vi "使用例子.vi"() -> ()   [LabVIEW 2015, in "PLC.lvlib"]
uses:
  PLC.lvlib
panel:
  in  "端口选择":refnum<visa-resource-name>="COM3"
  in  "波特率":u32(ring)=9600 items=["9600"=9600, "19200"=19200, "115200"=115200]
  in  "校检":u32(ring)=2 items=["无", "偶", "奇"]
  in  "数据位":u32(ring)=7 items=["7"=7, "8"=8]
  in  "16位/32位":u32(ring) items=["16bit", "32bit"]
  in  "写入":bool
  in  "写入数据":string
  in  "PLC地址":string="0"
  in  "变量类型":u32(ring)=2 items=["X", "Y", "M", "D"]
  out "读取数据输出":u32
  in  "读出":bool
  in  "M7":bool
  in  "M6":bool
  in  "M5":bool
  in  "M4":bool
  in  "M3":bool
  in  "M2":bool
  in  "M1":bool
  in  "M0":bool
  # "数据取值范围"
  # "寻址范围"
  # "X0-X577"
  # "0或1"
  # "Y0-Y577"
  # "0或1"
  # "M0-M7999"
  # "0或1"
  # "D0-D7999"
  # "16bit或32bit"
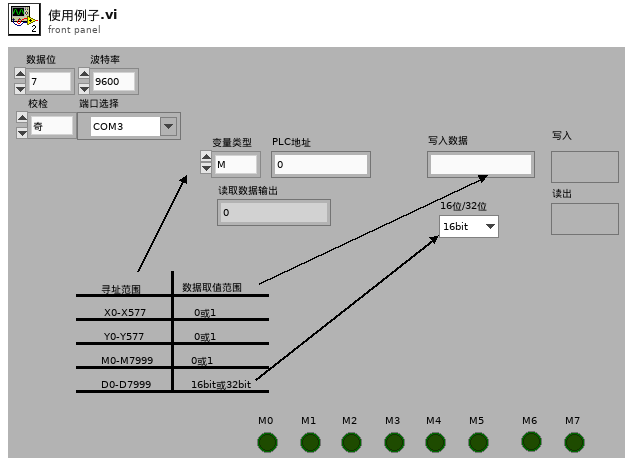
[diagram p1: front panel]
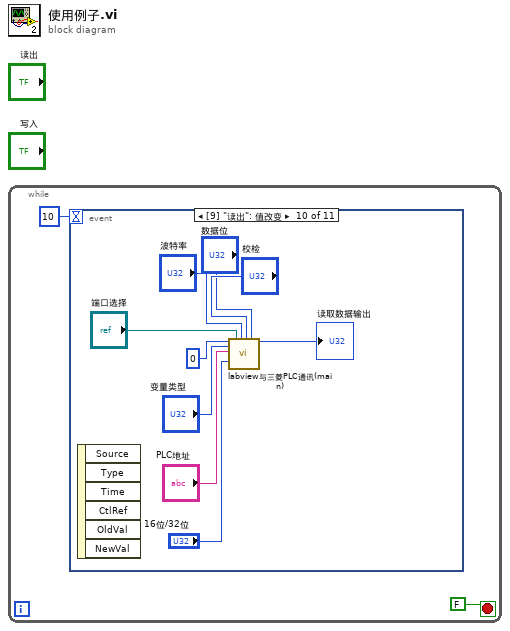
[diagram p0: block diagram]
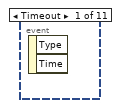
[diagram p2: hidden frame]
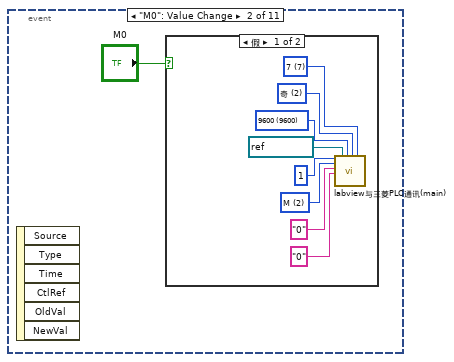
[diagram p3: hidden frame]
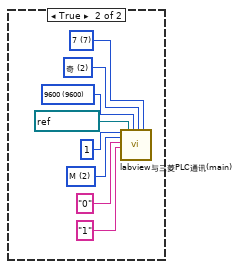
[diagram p4: hidden frame]
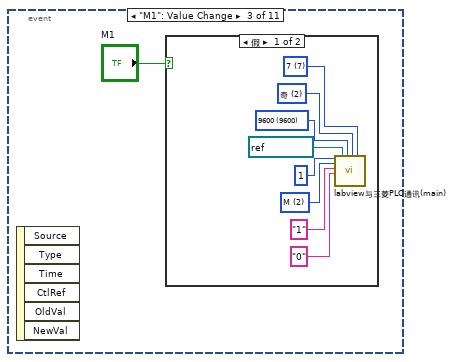
[diagram p5: hidden frame]
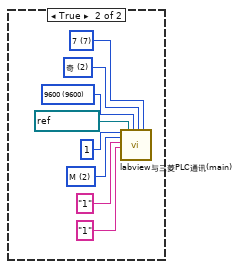
[diagram p6: hidden frame]
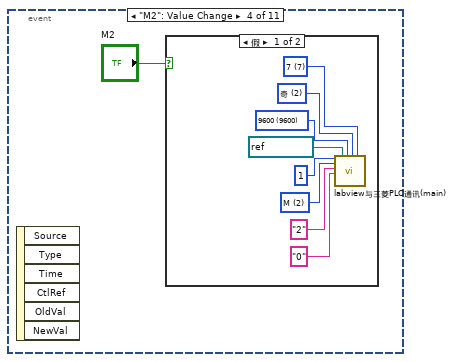
[diagram p7: hidden frame]
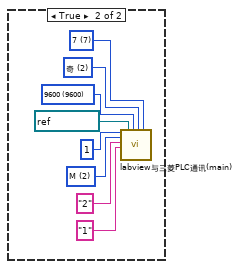
[diagram p8: hidden frame]
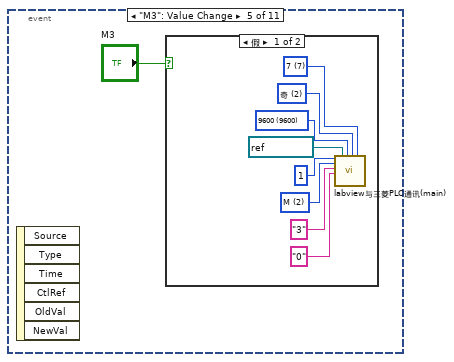
[diagram p9: hidden frame]
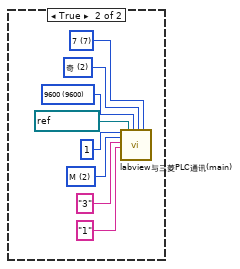
[diagram p10: hidden frame]
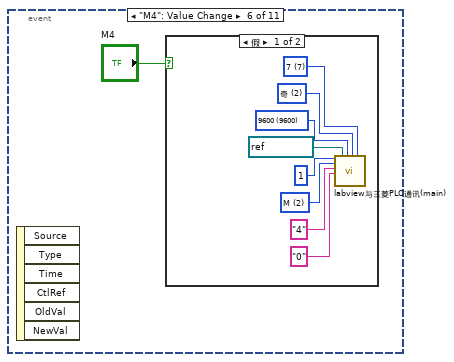
[diagram p11: hidden frame]
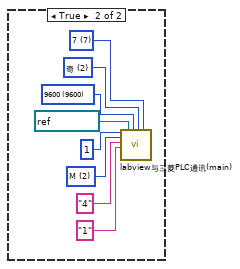
[diagram p12: hidden frame]
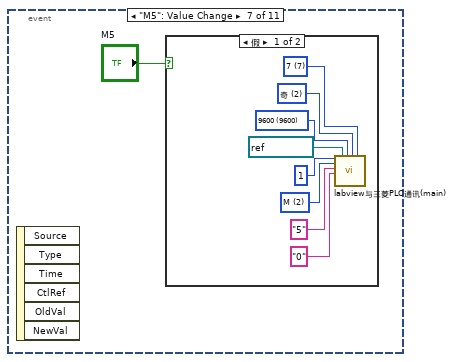
[diagram p13: hidden frame]
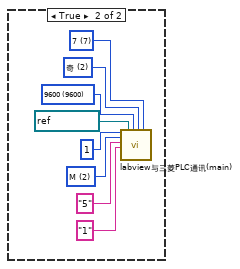
[diagram p14: hidden frame]
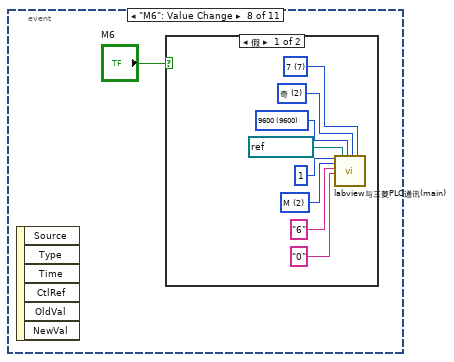
[diagram p15: hidden frame]
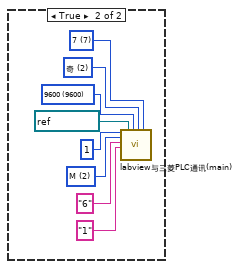
[diagram p16: hidden frame]
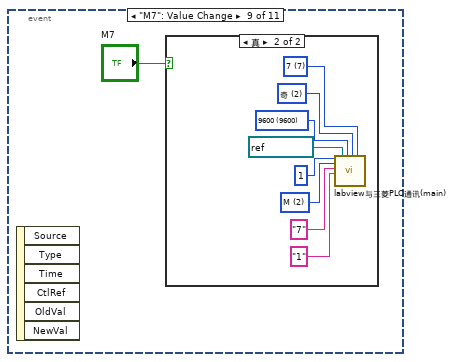
[diagram p17: hidden frame]
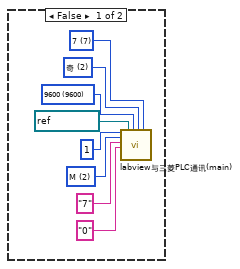
[diagram p18: hidden frame]
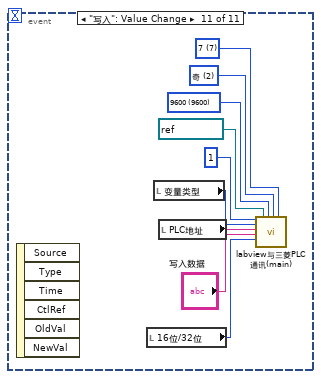
[diagram p19: hidden frame]
diagram:
  n1 = while {
    stop <- FALSE stop-if-true
    n2 = event shown="[9] \"读出\": 值改变" {
      selector: _ -> [_ _ _ _ _ _ _ _ _ _ _]
      dyn-events: _ -> [_ _ _ _ _ _ _ _ _ _ _]
      timeout: 10 -> [_ _ _ _ _ _ _ _ _ _ _]
      event Timeout {
        n3 = event-data() -> ()  [unwired: 3 out]
      }
      event "M0": Value Change {
        n4 = event-data() -> ()  [unwired: 7 out]
        n5 = case shown="假" "M0" {
          frame False {
            w6 = u32 2 items=["X", "Y", "M", "D"] ("变量类型")
            w8 = u32 7 items=["7"=7, "8"=8] ("数据位")
            w9 = u32 2 items=["无", "偶", "奇"] ("校检")
            w10 = u32 9600 items=["9600"=9600, "19200"=19200, "115200"=115200] ("波特率")
            n6 = call "labview与三菱PLC通讯(main).vi"("读取=0写入=1"=i16 1, "变量类型"=w6, "PLC地址"="0", "PLC数据"="0", "端口选择"=refnum<visa-resource-name> "COM3", "波特率"=w10, "校检"=w9, "数据位"=w8) -> ()  [unwired: 1 in, 11 out]
          }
          frame True {
            w14 = u32 2 items=["X", "Y", "M", "D"] ("变量类型")
            w16 = u32 7 items=["7"=7, "8"=8] ("数据位")
            w17 = u32 2 items=["无", "偶", "奇"] ("校检")
            w18 = u32 9600 items=["9600"=9600, "19200"=19200, "115200"=115200] ("波特率")
            n7 = call "labview与三菱PLC通讯(main).vi"("读取=0写入=1"=i16 1, "变量类型"=w14, "PLC地址"="0", "PLC数据"="1", "端口选择"=refnum<visa-resource-name> "COM3", "波特率"=w18, "校检"=w17, "数据位"=w16) -> ()  [unwired: 1 in, 11 out]
          }
        }
      }
      event "M1": Value Change {
        n8 = event-data() -> ()  [unwired: 7 out]
        n9 = case shown="假" "M1" {
          frame False {
            w23 = u32 2 items=["X", "Y", "M", "D"] ("变量类型")
            w25 = u32 7 items=["7"=7, "8"=8] ("数据位")
            w26 = u32 2 items=["无", "偶", "奇"] ("校检")
            w27 = u32 9600 items=["9600"=9600, "19200"=19200, "115200"=115200] ("波特率")
            n10 = call "labview与三菱PLC通讯(main).vi"("读取=0写入=1"=i16 1, "变量类型"=w23, "PLC地址"="1", "PLC数据"="0", "端口选择"=refnum<visa-resource-name> "COM3", "波特率"=w27, "校检"=w26, "数据位"=w25) -> ()  [unwired: 1 in, 11 out]
          }
          frame True {
            w31 = u32 2 items=["X", "Y", "M", "D"] ("变量类型")
            w33 = u32 7 items=["7"=7, "8"=8] ("数据位")
            w34 = u32 2 items=["无", "偶", "奇"] ("校检")
            w35 = u32 9600 items=["9600"=9600, "19200"=19200, "115200"=115200] ("波特率")
            n11 = call "labview与三菱PLC通讯(main).vi"("读取=0写入=1"=i16 1, "变量类型"=w31, "PLC地址"="1", "PLC数据"="1", "端口选择"=refnum<visa-resource-name> "COM3", "波特率"=w35, "校检"=w34, "数据位"=w33) -> ()  [unwired: 1 in, 11 out]
          }
        }
      }
      event "M2": Value Change {
        n12 = event-data() -> ()  [unwired: 7 out]
        n13 = case shown="假" "M2" {
          frame False {
            w40 = u32 2 items=["X", "Y", "M", "D"] ("变量类型")
            w42 = u32 7 items=["7"=7, "8"=8] ("数据位")
            w43 = u32 2 items=["无", "偶", "奇"] ("校检")
            w44 = u32 9600 items=["9600"=9600, "19200"=19200, "115200"=115200] ("波特率")
            n14 = call "labview与三菱PLC通讯(main).vi"("读取=0写入=1"=i16 1, "变量类型"=w40, "PLC地址"="2", "PLC数据"="0", "端口选择"=refnum<visa-resource-name> "COM3", "波特率"=w44, "校检"=w43, "数据位"=w42) -> ()  [unwired: 1 in, 11 out]
          }
          frame True {
            w48 = u32 2 items=["X", "Y", "M", "D"] ("变量类型")
            w50 = u32 7 items=["7"=7, "8"=8] ("数据位")
            w51 = u32 2 items=["无", "偶", "奇"] ("校检")
            w52 = u32 9600 items=["9600"=9600, "19200"=19200, "115200"=115200] ("波特率")
            n15 = call "labview与三菱PLC通讯(main).vi"("读取=0写入=1"=i16 1, "变量类型"=w48, "PLC地址"="2", "PLC数据"="1", "端口选择"=refnum<visa-resource-name> "COM3", "波特率"=w52, "校检"=w51, "数据位"=w50) -> ()  [unwired: 1 in, 11 out]
          }
        }
      }
      event "M3": Value Change {
        n16 = event-data() -> ()  [unwired: 7 out]
        n17 = case shown="假" "M3" {
          frame False {
            w57 = u32 2 items=["X", "Y", "M", "D"] ("变量类型")
            w59 = u32 7 items=["7"=7, "8"=8] ("数据位")
            w60 = u32 2 items=["无", "偶", "奇"] ("校检")
            w61 = u32 9600 items=["9600"=9600, "19200"=19200, "115200"=115200] ("波特率")
            n18 = call "labview与三菱PLC通讯(main).vi"("读取=0写入=1"=i16 1, "变量类型"=w57, "PLC地址"="3", "PLC数据"="0", "端口选择"=refnum<visa-resource-name> "COM3", "波特率"=w61, "校检"=w60, "数据位"=w59) -> ()  [unwired: 1 in, 11 out]
          }
          frame True {
            w65 = u32 2 items=["X", "Y", "M", "D"] ("变量类型")
            w67 = u32 7 items=["7"=7, "8"=8] ("数据位")
            w68 = u32 2 items=["无", "偶", "奇"] ("校检")
            w69 = u32 9600 items=["9600"=9600, "19200"=19200, "115200"=115200] ("波特率")
            n19 = call "labview与三菱PLC通讯(main).vi"("读取=0写入=1"=i16 1, "变量类型"=w65, "PLC地址"="3", "PLC数据"="1", "端口选择"=refnum<visa-resource-name> "COM3", "波特率"=w69, "校检"=w68, "数据位"=w67) -> ()  [unwired: 1 in, 11 out]
          }
        }
      }
      event "M4": Value Change {
        n20 = event-data() -> ()  [unwired: 7 out]
        n21 = case shown="假" "M4" {
          frame False {
            w74 = u32 2 items=["X", "Y", "M", "D"] ("变量类型")
            w76 = u32 7 items=["7"=7, "8"=8] ("数据位")
            w77 = u32 2 items=["无", "偶", "奇"] ("校检")
            w78 = u32 9600 items=["9600"=9600, "19200"=19200, "115200"=115200] ("波特率")
            n22 = call "labview与三菱PLC通讯(main).vi"("读取=0写入=1"=i16 1, "变量类型"=w74, "PLC地址"="4", "PLC数据"="0", "端口选择"=refnum<visa-resource-name> "COM3", "波特率"=w78, "校检"=w77, "数据位"=w76) -> ()  [unwired: 1 in, 11 out]
          }
          frame True {
            w82 = u32 2 items=["X", "Y", "M", "D"] ("变量类型")
            w84 = u32 7 items=["7"=7, "8"=8] ("数据位")
            w85 = u32 2 items=["无", "偶", "奇"] ("校检")
            w86 = u32 9600 items=["9600"=9600, "19200"=19200, "115200"=115200] ("波特率")
            n23 = call "labview与三菱PLC通讯(main).vi"("读取=0写入=1"=i16 1, "变量类型"=w82, "PLC地址"="4", "PLC数据"="1", "端口选择"=refnum<visa-resource-name> "COM3", "波特率"=w86, "校检"=w85, "数据位"=w84) -> ()  [unwired: 1 in, 11 out]
          }
        }
      }
      event "M5": Value Change {
        n24 = event-data() -> ()  [unwired: 7 out]
        n25 = case shown="假" "M5" {
          frame False {
            w91 = u32 2 items=["X", "Y", "M", "D"] ("变量类型")
            w93 = u32 7 items=["7"=7, "8"=8] ("数据位")
            w94 = u32 2 items=["无", "偶", "奇"] ("校检")
            w95 = u32 9600 items=["9600"=9600, "19200"=19200, "115200"=115200] ("波特率")
            n26 = call "labview与三菱PLC通讯(main).vi"("读取=0写入=1"=i16 1, "变量类型"=w91, "PLC地址"="5", "PLC数据"="0", "端口选择"=refnum<visa-resource-name> "COM3", "波特率"=w95, "校检"=w94, "数据位"=w93) -> ()  [unwired: 1 in, 11 out]
          }
          frame True {
            w99 = u32 2 items=["X", "Y", "M", "D"] ("变量类型")
            w101 = u32 7 items=["7"=7, "8"=8] ("数据位")
            w102 = u32 2 items=["无", "偶", "奇"] ("校检")
            w103 = u32 9600 items=["9600"=9600, "19200"=19200, "115200"=115200] ("波特率")
            n27 = call "labview与三菱PLC通讯(main).vi"("读取=0写入=1"=i16 1, "变量类型"=w99, "PLC地址"="5", "PLC数据"="1", "端口选择"=refnum<visa-resource-name> "COM3", "波特率"=w103, "校检"=w102, "数据位"=w101) -> ()  [unwired: 1 in, 11 out]
          }
        }
      }
      event "M6": Value Change {
        n28 = event-data() -> ()  [unwired: 7 out]
        n29 = case shown="假" "M6" {
          frame False {
            w108 = u32 2 items=["X", "Y", "M", "D"] ("变量类型")
            w110 = u32 7 items=["7"=7, "8"=8] ("数据位")
            w111 = u32 2 items=["无", "偶", "奇"] ("校检")
            w112 = u32 9600 items=["9600"=9600, "19200"=19200, "115200"=115200] ("波特率")
            n30 = call "labview与三菱PLC通讯(main).vi"("读取=0写入=1"=i16 1, "变量类型"=w108, "PLC地址"="6", "PLC数据"="0", "端口选择"=refnum<visa-resource-name> "COM3", "波特率"=w112, "校检"=w111, "数据位"=w110) -> ()  [unwired: 1 in, 11 out]
          }
          frame True {
            w116 = u32 2 items=["X", "Y", "M", "D"] ("变量类型")
            w118 = u32 7 items=["7"=7, "8"=8] ("数据位")
            w119 = u32 2 items=["无", "偶", "奇"] ("校检")
            w120 = u32 9600 items=["9600"=9600, "19200"=19200, "115200"=115200] ("波特率")
            n31 = call "labview与三菱PLC通讯(main).vi"("读取=0写入=1"=i16 1, "变量类型"=w116, "PLC地址"="6", "PLC数据"="1", "端口选择"=refnum<visa-resource-name> "COM3", "波特率"=w120, "校检"=w119, "数据位"=w118) -> ()  [unwired: 1 in, 11 out]
          }
        }
      }
      event "M7": Value Change {
        n32 = event-data() -> ()  [unwired: 7 out]
        n33 = case shown="真" "M7" {
          frame False {
            w125 = u32 2 items=["X", "Y", "M", "D"] ("变量类型")
            w127 = u32 7 items=["7"=7, "8"=8] ("数据位")
            w128 = u32 2 items=["无", "偶", "奇"] ("校检")
            w129 = u32 9600 items=["9600"=9600, "19200"=19200, "115200"=115200] ("波特率")
            n34 = call "labview与三菱PLC通讯(main).vi"("读取=0写入=1"=i16 1, "变量类型"=w125, "PLC地址"="7", "PLC数据"="0", "端口选择"=refnum<visa-resource-name> "COM3", "波特率"=w129, "校检"=w128, "数据位"=w127) -> ()  [unwired: 1 in, 11 out]
          }
          frame True {
            w133 = u32 2 items=["X", "Y", "M", "D"] ("变量类型")
            w135 = u32 7 items=["7"=7, "8"=8] ("数据位")
            w136 = u32 2 items=["无", "偶", "奇"] ("校检")
            w137 = u32 9600 items=["9600"=9600, "19200"=19200, "115200"=115200] ("波特率")
            n35 = call "labview与三菱PLC通讯(main).vi"("读取=0写入=1"=i16 1, "变量类型"=w133, "PLC地址"="7", "PLC数据"="1", "端口选择"=refnum<visa-resource-name> "COM3", "波特率"=w137, "校检"=w136, "数据位"=w135) -> ()  [unwired: 1 in, 11 out]
          }
        }
      }
      event "读出": Value Change {
        n36 = event-data() -> ()  [unwired: 7 out]
        n37 = call "labview与三菱PLC通讯(main).vi"("读取=0写入=1"=i16 0, "变量类型"="变量类型", "PLC地址"="PLC地址", "16位/32位"="16位/32位", "端口选择"="端口选择", "波特率"="波特率", "校检"="校检", "数据位"="数据位") -> ("读取数据输出"=→"读取数据输出":u32)  [unwired: 1 in, 10 out]
      }
      event "写入": Value Change {
        w153 = u32 7 items=["7"=7, "8"=8] ("数据位")
        w154 = u32 2 items=["无", "偶", "奇"] ("校检")
        w155 = u32 9600 items=["9600"=9600, "19200"=19200, "115200"=115200] ("波特率")
        n38 = event-data() -> ()  [unwired: 7 out]
        n39 = local read "16位/32位"() -> (w148:u32)
        n40 = local read "变量类型"() -> (w150:u32)
        n41 = local read "PLC地址"() -> (w149:string)
        n42 = call "labview与三菱PLC通讯(main).vi"("读取=0写入=1"=i16 1, "变量类型"=w150, "PLC地址"=w149, "PLC数据"="写入数据", "16位/32位"=w148, "端口选择"=refnum<visa-resource-name> "COM3", "波特率"=w155, "校检"=w154, "数据位"=w153) -> ()  [unwired: 11 out]
      }
    }
  }
